vi "AlazarGetWhotriggeredBySystemID.vi"(3 "error in (no error)":errorcluster, 4 "Record Number":u32, 5 "Board ID":u32, 6 "System ID":u32) -> (0 "error out":errorcluster, 2 "Who":u32(ring) items=["Not this board", "Channel A", "Channel B", "Ext. Trig. In", "Ch. A and ch. B", "Ch. A and Ext. Trig. In.", "Ch. B and Ext. Trig. In.", "Trigger Timeout"])   [LabVIEW 2009]
doc: "Return which event caused a board system to trigger and capture a record to on-board memory."
uses:
  ATSApi.dll
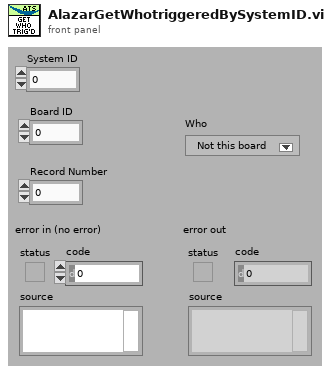
[diagram p1: front panel]
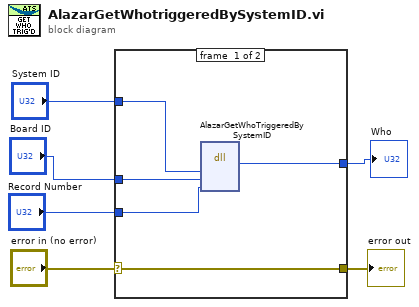
[diagram p0: block diagram]
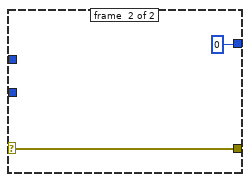
[diagram p2: hidden frame]
diagram:
  n1 = case shown="No Error" "error in (no error)" {
    selector: "error in (no error)" -> [w10 w13]
    tunnel: [w10 w13] -> w5
    tunnel: "System ID" -> [w11 _]
    tunnel: "Board ID" -> [w9 _]
    tunnel: "Record Number" -> [w8 _]
    tunnel: [w7 u32 0] -> w1
    frame #0 {
      n2 = dll-call lib="ATSApi.dll" fn="AlazarGetWhoTriggeredBySystemID"("systemId"=w11, "boardID"=w9, "recordNumber"=w8) -> (w7:u32)  [unwired: 6 in, 2 out]
    }
    frame #1 {
    }
  }
  "error out" <- w5
  "Who" <- w1
